vi "Clamp AET Min_Vertical_shan.vi"(6 "Edge Options":T4={"Edge Polarity"=0, "Kernel Size"=3, "Width"=3, "Minimum Edge Strength"=10.0, "Interpolation Type"=enum."Bilinear Fixed", "Data Processing Method"=enum."Average"} {"Edge Polarity" items=["All Edges", "Rising Edges", "Falling Edges"]; "Minimum Edge Strength" format="%.2f"; "Width" step=2; "Kernel Size" step=2}, 7 "Scanning axis":u16(ring)=1 items=["Left To Right", "Right To Left", "Top To Bottom", "Bottom To Top"], 8 "error in (no error)":errorcluster, 9 "Coordinate System":T8 {"Measurement System"."Axis Reference" items=["Direct", "Indirect"]; "Measurement System"."Angle (deg)" format="%.2f"; "Measurement System"."Origin"."Y" format="%.2f"; "Measurement System"."Origin"."X" format="%.2f"; "Reference System"."Axis Reference" items=["Direct", "Indirect"]; "Reference System"."Angle (deg)" format="%.2f"; "Reference System"."Origin"."Y" format="%.2f"; "Reference System"."Origin"."X" format="%.2f"}, 10 "ROI Descriptor":T1 {"Contours"."Type" items=["No Selection", "Point", "Line", "Rectangle", "Oval", "Polygon", "Freehand Region", "Annulus", "Unused2", "Unused3", "Broken Line", "Freehand Line", "Rotated Rectangle"]}, 11 "Image":T7) -> (0 "error out":errorcluster, 1 "Coordinate System (duplicate)":T8 {"Measurement System"."Axis Reference" items=["Direct", "Indirect"]; "Measurement System"."Angle (deg)" format="%.2f"; "Measurement System"."Origin"."Y" format="%.2f"; "Measurement System"."Origin"."X" format="%.2f"; "Reference System"."Axis Reference" items=["Direct", "Indirect"]; "Reference System"."Angle (deg)" format="%.2f"; "Reference System"."Origin"."Y" format="%.2f"; "Reference System"."Origin"."X" format="%.2f"}, 2 "Distance":sgl format="%.2f", 3 "Image Out":T7, 4 "Perpendicular Lines":T2(array[cluster])=[{{"X"=55.0, "Y"=48.0}, {"X"=263.0, "Y"=104.0}}, {{"X"=53.0, "Y"=53.0}, {"X"=262.0, "Y"=109.0}}, {{"X"=52.0, "Y"=58.0}, {"X"=261.0, "Y"=113.0}}, {{"X"=51.0, "Y"=62.0}, {"X"=259.0, "Y"=118.0}}, {{"X"=49.0, "Y"=67.0}, {"X"=258.0, "Y"=123.0}}, {{"X"=48.0, "Y"=72.0}, {"X"=257.0, "Y"=128.0}}, {{"X"=47.0, "Y"=77.0}, {"X"=255.0, "Y"=133.0}}, {{"X"=46.0, "Y"=82.0}, {"X"=254.0, "Y"=138.0}}, {{"X"=44.0, "Y"=87.0}, {"X"=253.0, "Y"=142.0}}, {{"X"=43.0, "Y"=91.0}, {"X"=252.0, "Y"=147.0}}, {{"X"=42.0, "Y"=96.0}, {"X"=250.0, "Y"=152.0}}] {"?"."Y" format="%.2f"; "?"."X" format="%.2f"; "?"."Y" format="%.2f"; "?"."X" format="%.2f"}, 5 "Edge Coordinates":cluster{"X":sgl, "Y":sgl}[](array[cluster]) {"Y" format="%.2f"; "X" format="%.2f"})   [LabVIEW 2015]
doc: "Modified NI Vertical Max Clamp with Rake-3 which uses Advanced Edge Detection."
uses:
  <vilib>/vision/Image Controls.llb/IMAQ Image.ctl
  <vilib>/vision/Measure.llb/Edge Options.ctl
  <vilib>/vision/Measure.llb/Edge Polarity.ctl
  <vilib>/vision/NI_Vision_Development_Module.lvlib
panel:
  in  "Rect for the clamp":T3 {"Rotation" format="%.2f"; "Left" scale=0.0..1024.0; "Right" scale=0.0..1024.0}
  in  "Settings":T6={"Contrast"=50, "Filter width"=4, "Steepness"=2, "Subsampling Ratio"=5, "Show Search Area"=FALSE, "Show Search Lines"=FALSE, "Show Edges Found"=FALSE, "Show Result"=TRUE}
  out "Elapsed time (ms)":u32
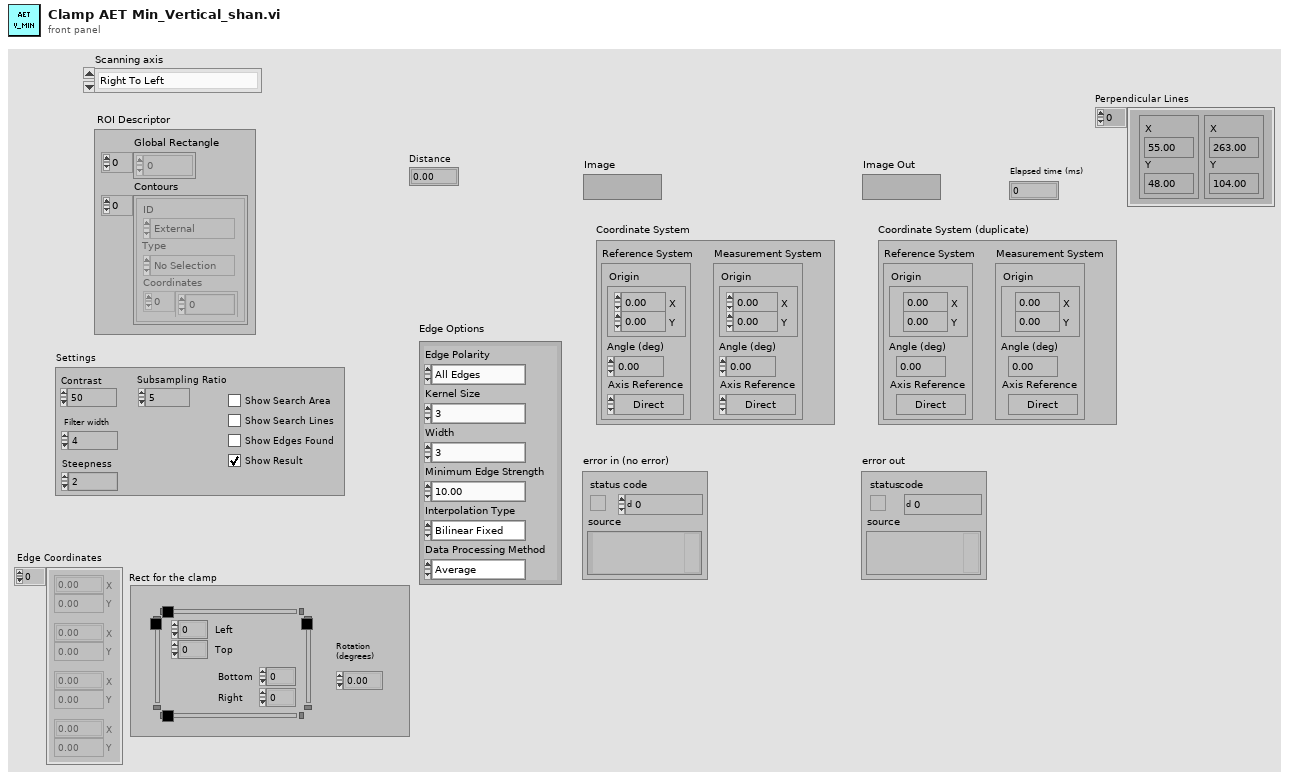
[diagram p1: front panel]
types:
  T1 = typedef "ROI Descriptor" = cluster{"Global Rectangle":i32[], "Contours":cluster{"ID":enum32{"External", "Internal"}, "Type":u32, "Coordinates":i32[]}[]}
  T2 = cluster{cluster{"X":sgl, "Y":sgl}, cluster{"X":sgl, "Y":sgl}}[]
  T3 = typedef "IMAQ Rectangle" = cluster{"Left":i32, "Top":i32, "Right":i32, "Bottom":i32, "Rotation":dbl}
  T4 = typedef "Edge Options.ctl" = cluster{"Edge Polarity":T5, "Kernel Size":u32, "Width":u32, "Minimum Edge Strength":sgl, "Interpolation Type":enum32{"Zero Order", "Bilinear", "Quadratic", "Cubic", "Bilinear Fixed"}, "Data Processing Method":enum32{"Average", "Median"}}
  T5 = typedef "Edge Polarity.ctl" = u32
  T6 = cluster{"Contrast":i32, "Filter width":i32, "Steepness":i32, "Subsampling Ratio":u32, "Show Search Area":bool, "Show Search Lines":bool, "Show Edges Found":bool, "Show Result":bool}
  T7 = typedef "IMAQ Image.ctl" = refnum<image>
  T8 = typedef "IMAQ Coordinate System" = cluster{"Reference System":cluster{"Origin":cluster{"X":sgl, "Y":sgl}, "Angle (deg)":sgl, "Axis Reference":u32}, "Measurement System":cluster{"Origin":cluster{"X":sgl, "Y":sgl}, "Angle (deg)":sgl, "Axis Reference":u32}}
  T9 = enum16{"Get First Edge", "Get First + Last Edge", "Get All Edges", "Get Best Edge"}
  T10 = cluster{"Start Point":cluster{"X":sgl, "Y":sgl}, "End Point":cluster{"X":sgl, "Y":sgl}}
  T11 = typedef "Edge New.ctl" = cluster{"Location (Pixel)":cluster{"X":sgl, "Y":sgl}, "Location (Real-World)":cluster{"X":sgl, "Y":sgl}, "Distance (Pixel)":dbl, "Distance (Real-World)":dbl, "Strength":dbl, "Noise":dbl, "Rising?":bool}
  T12 = typedef "Search Line.ctl" = cluster{"Start Point":cluster{"X":sgl, "Y":sgl}, "End Point":cluster{"X":sgl, "Y":sgl}, "Edge Info":T11[], "Edge Map":dbl[], "Calibration Valid":bool}
  T13 = cluster{"Show Search Area":bool, "Show Search Lines":bool, "Show Edges Found":bool, "Show Result":bool}
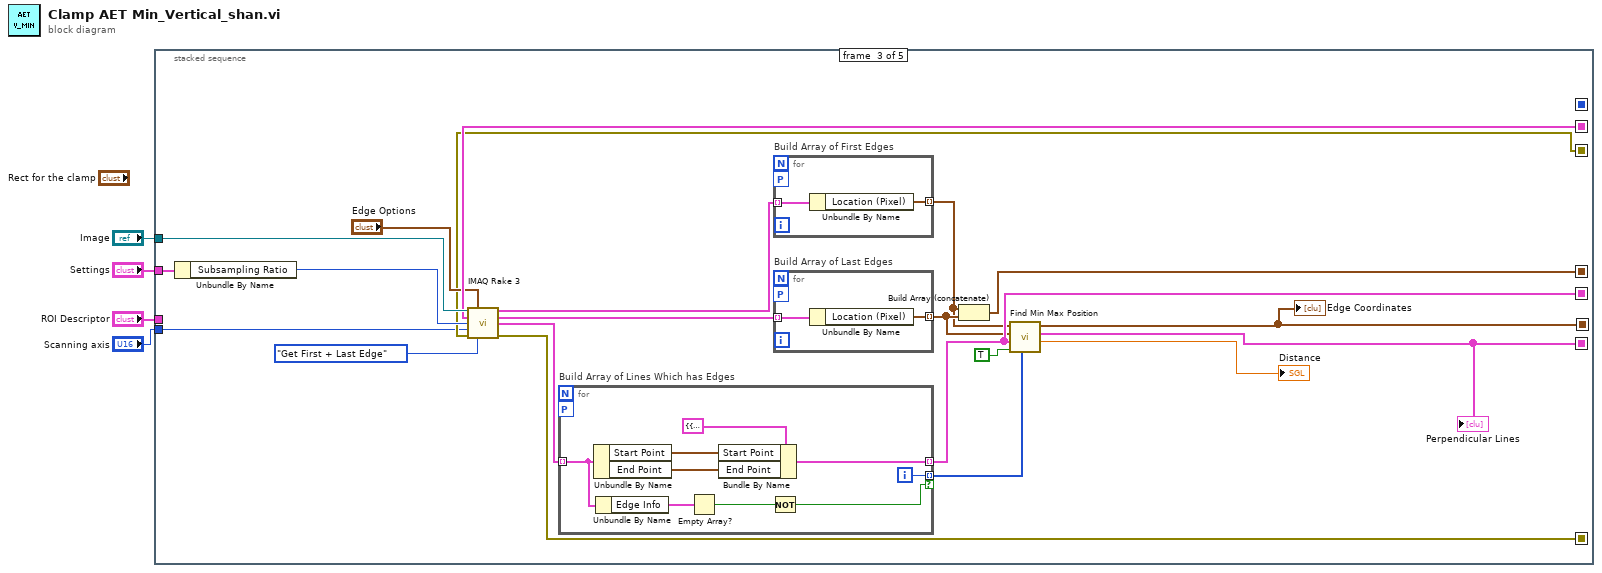
[diagram p0: block diagram]
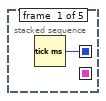
[diagram p2: hidden frame]
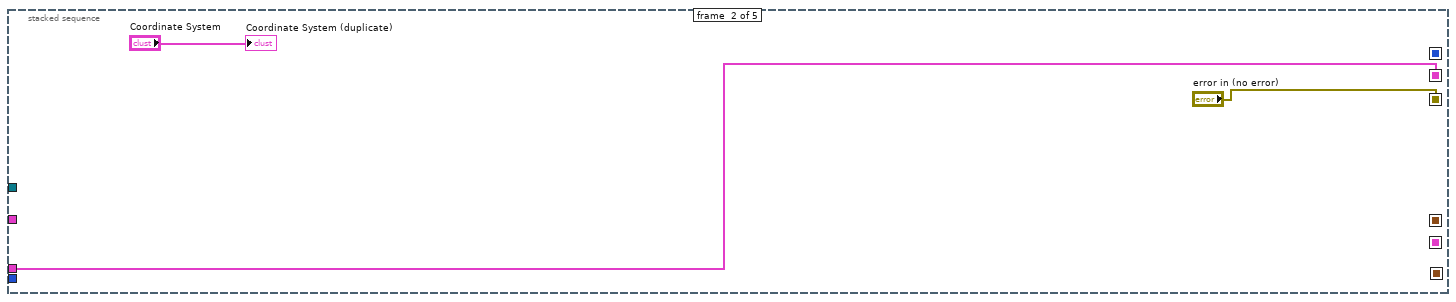
[diagram p3: hidden frame]
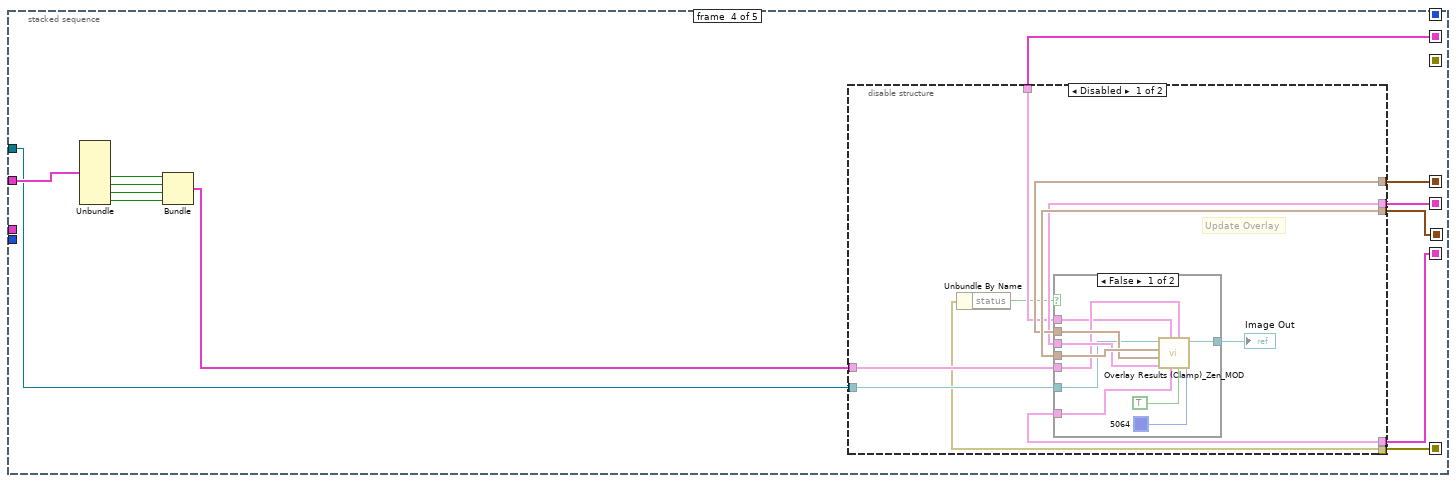
[diagram p4: hidden frame]
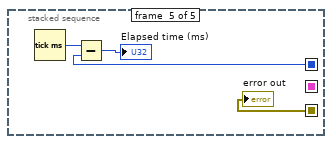
[diagram p7: hidden frame]
diagram:
  n1 = stacked-sequence {
    seq-local: [_ _ w18 _ _] -> [_ _ _ w55 _]
    seq-local: [w5 _ _ _ _] -> [_ _ _ _ w80]
    seq-local: [_ _ w20 _ _] -> [_ _ _ w54 _]
    seq-local: [_ _ w22 _ _] -> [_ _ _ w53 _]
    seq-local: [_ _ w19 _ _] -> [_ _ _ w47 _]
    seq-local: [_ w6 _ _ _] -> [_ _ w27 w45 _]
    seq-local: [_ "error in (no error)" _ _ _] -> [_ _ w13 _ w77]
    seq-local: [_ _ w12 _ _] -> [_ _ _ w43 _]
    tunnel: "Image" -> [_ _ w28 w44 _]
    tunnel: "Settings" -> [_ _ w29 w52 _]
    tunnel: "ROI Descriptor" -> [_ w6 _ _ _]
    tunnel: "Scanning axis" -> [_ _ w9 _ _]
    frame #0 {
      n2 = Tick Count (ms)() -> (millisecond timer value=w5:u32)
    }
    frame #1 {
      "Coordinate System (duplicate)" <- "Coordinate System"
    }
    frame #2 {
      n3 = Unbundle By Name(w29) -> ("Subsampling Ratio"=w26:u32)
      n4 = call "IMAQ Rake 3"("Image"=w28, "Edge Options"="Edge Options", "ROI Descriptor"=w27, "Step Size"=w26, "Scan Direction"=w9, "error in (no error)"=w13, "Process"=T9."Get First + Last Edge") -> ("First Edges"=w24:T11[], "Last Edges"=w23:T11[], "Search Lines"=w11:T12[], "error out"=w12:errorcluster)  [unwired: 5 in]
      n5 = for "Build Array of Lines Which has Edges" {
        tunnel: w11 -> [w35] mode=indexing
        tunnel: [w36] -> w22 mode=indexing
        tunnel: [w32] -> w15 mode=indexing if=w31
        workers-P: _ -> [_]
        i -> [w32]
        n6 = Unbundle By Name(w35) -> ("Start Point"=w38:cluster{"X":sgl, "Y":sgl}, "End Point"=w37:cluster{"X":sgl, "Y":sgl})
        n7 = Unbundle By Name(w35) -> ("Edge Info"=w34:T11[])
        n8 = Empty Array?(array=w34) -> (empty?=w33:bool)
        n9 = Bundle By Name(cluster=T10 {"Start Point"={"X"=0.0, "Y"=0.0}, "End Point"={"X"=0.0, "Y"=0.0}} ("Cluster 2"), "Start Point"=w38, "End Point"=w37) -> (w36:T10)
        n10 = Not(x=w33) -> (.not. x?=w31:bool)
      }
      n11 = for "Build Array of First Edges" {
        tunnel: w24 -> [w42] mode=indexing
        tunnel: [w41] -> w16 mode=indexing
        workers-P: _ -> [_]
        n12 = Unbundle By Name(w42) -> ("Location (Pixel)"=w41:cluster{"X":sgl, "Y":sgl})
      }
      n13 = for "Build Array of Last Edges" {
        tunnel: w23 -> [w40] mode=indexing
        tunnel: [w39] -> w21 mode=indexing
        workers-P: _ -> [_]
        n14 = Unbundle By Name(w40) -> ("Location (Pixel)"=w39:cluster{"X":sgl, "Y":sgl})
      }
      n15 = Build Array (concatenate)(w16, w21) -> (w20:cluster{"X":sgl, "Y":sgl}[])
      n16 = call <vilib>:"Find Min Max Position.vi"("Lines with Edges (first)"=w15, "Min / Max"=TRUE, "Search Lines"=w22, "Last Edges"=w21, "First Edges"=w16) -> ("Distance"=→"Distance":sgl, "Perpendicular Lines"=w19:T2, "Points"=w18:cluster{"X":sgl, "Y":sgl}[])  [unwired: 1 in, 3 out]
      "Edge Coordinates" <- w18
      "Perpendicular Lines" <- w19
    }
    frame #3 {
      n17 = Unbundle(w52) -> ("Show Search Area"=w51:bool, "Show Search Lines"=w50:bool, "Show Edges Found"=w49:bool, "Show Result"=w48:bool)  [unwired: 4 out]
      n18 = Bundle("Show Search Area"=w51, "Show Search Lines"=w50, "Show Edges Found"=w49, "Show Result"=w48) -> (w46:T13)  [unwired: 1 out]
      n19 = disable-structure shown="Disabled" {
        disable-tunnel: w55 -> [w65 _]
        disable-tunnel: w54 -> [w64 _]
        disable-tunnel: w53 -> [w63 _]
        disable-tunnel: w47 -> [w62 _]
        disable-tunnel: w46 -> [w61 _]
        disable-tunnel: w45 -> [w60 _]
        disable-tunnel: w44 -> [w59 _]
        disable-tunnel: w43 -> [w56 _]
        frame Disabled {
          # "Update Overlay"
          n20 = Unbundle By Name(w56) -> ("status"=w57:bool)
          n21 = case shown="False" w57 {
            tunnel: w65 -> [w75 _]
            tunnel: w64 -> [w74 _]
            tunnel: w63 -> [w73 _]
            tunnel: w62 -> [w72 _]
            tunnel: w61 -> [w70 _]
            tunnel: w60 -> [w69 _]
            tunnel: w59 -> [w68 w76]
            tunnel: [w67 w76] -> w58
            frame False {
              n22 = call "Overlay Results (Clamp)_Zen_MOD.vi"("Result Color"=u32 5064, "Min / Max"=TRUE, "Setup"=w70, "Perpendicular Lines"=w72, "ROI Descriptor"=w69, "Search Lines"=w73, "All Edges Found"=w74, "Measurement Edges"=w75, "Image In"=w68) -> ("Image Out"=w67:T7)  [unwired: 2 in]
            }
            frame True {
            }
          }
          "Image Out" <- w58
        }
        frame Enabled {
        }
      }
    }
    frame #4 {
      n23 = Tick Count (ms)() -> (millisecond timer value=w79:u32)
      n24 = Subtract(x=w79, y=w80) -> (x-y=→"Elapsed time (ms)":u32)
      "error out" <- w77
    }
  }
